vi "Start Tx.vi"(3 "error in (no error)":errorcluster, 5 "Cluster":T1) -> (0 "error out":errorcluster)   [LabVIEW 2015, in "QCA_DUT_Func.lvlib"]
doc: "DLL_QMSL_AEROFLEX void _stdcall StartTx(int txMode,int channel,int rateBitIndex0,int wlanMode,int pktLen0,int txChain0,int shortGuard,int numPackets,int broadcast,int flags,int gainIdx,int dacGain,int paConfig,int tpcm);"
uses:
  QCA_DUT_Func.lvlib
  QCA_DUT_Func.dll
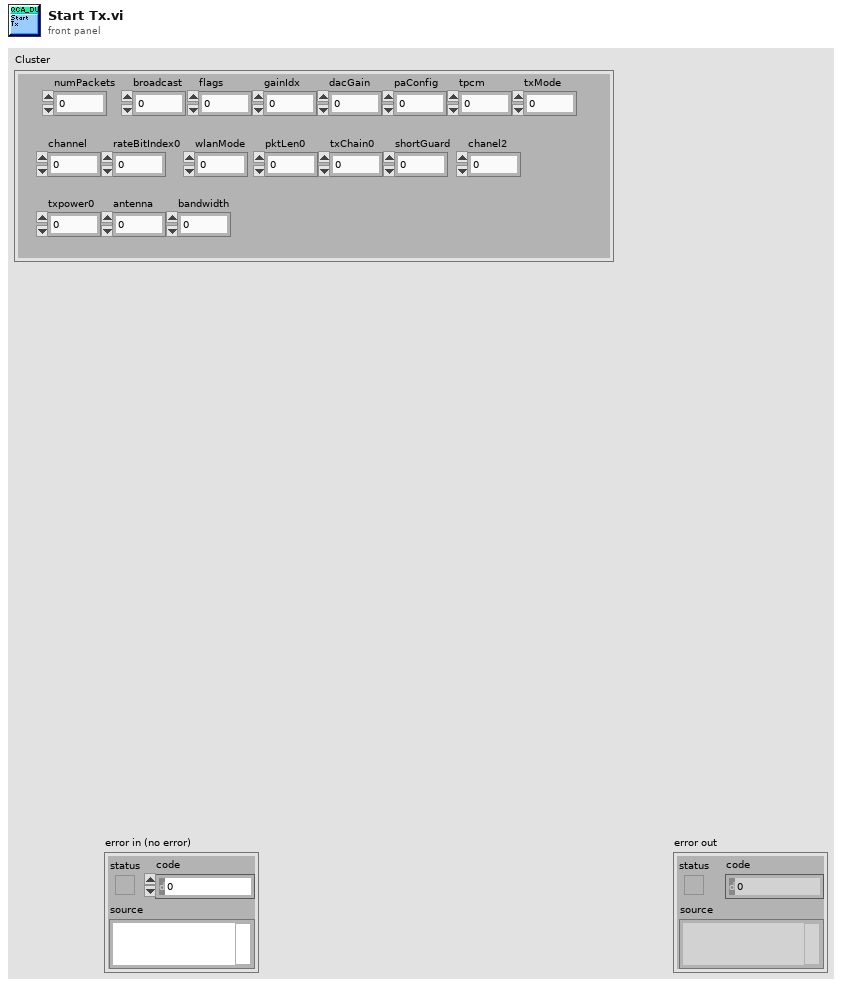
[diagram p1: front panel]
types:
  T1 = cluster{"numPackets":i32, "broadcast":i32, "flags":i32, "gainIdx":i32, "dacGain":i32, "paConfig":i32, "tpcm":i32, "txMode":i32, "channel":i32, "rateBitIndex0":i32, "wlanMode":i32, "pktLen0":i32, "txChain0":i32, "shortGuard":i32, "chanel2":i32, "txpower0":dbl, "antenna":i32, "bandwidth":i32}
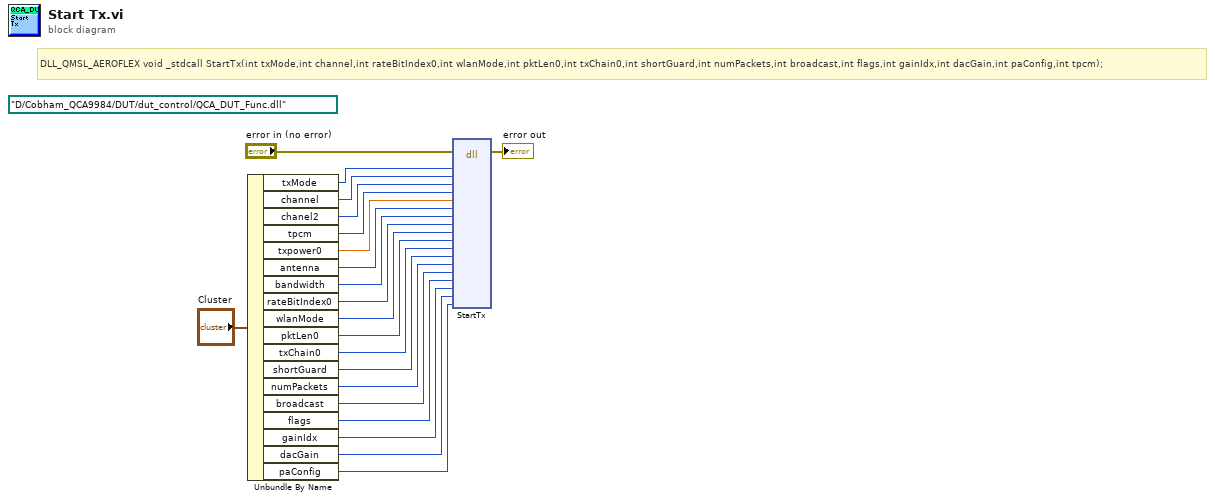
[diagram p0: block diagram]
diagram:
  (unwired) path "D:/Cobham_QCA9984/DUT/dut_control/QCA_DUT_Func.dll" ("path in")
  # "DLL_QMSL_AEROFLEX void _stdcall StartTx(int txMode,int channel,int rateBitIndex0,int wlanMode,int pktLen0,int txChain0,int shortGuard,int numPackets,int broadcast,int flags,int gainIdx,int dacGain,int paConfig,int tpcm);"
  n1 = Unbundle By Name("Cluster") -> ("txMode"=w18:i32, "channel"=w17:i32, "chanel2"=w16:i32, "tpcm"=w15:i32, "txpower0"=w14:dbl, "antenna"=w13:i32, "bandwidth"=w12:i32, "rateBitIndex0"=w11:i32, "wlanMode"=w10:i32, "pktLen0"=w9:i32, "txChain0"=w8:i32, "shortGuard"=w7:i32, "numPackets"=w6:i32, "broadcast"=w5:i32, "flags"=w4:i32, "gainIdx"=w3:i32, "dacGain"=w2:i32, "paConfig"=w1:i32)
  n2 = dll-call lib="D:/4-Up-WLAN-Test-System/DUT Control/DUT/dut_control/QCA_DUT_Func.dll" fn="StartTx"(error in="error in (no error)", "txMode"=w18, "channel"=w17, "chanel2"=w16, "tpcm"=w15, "txpower0"=w14, "antenna"=w13, "bandwidth"=w12, "rateBitIndex0"=w11, "wlanMode"=w10, "pktLen0"=w9, "txChain0"=w8, "shortGuard"=w7, "numPackets"=w6, "broadcast"=w5, "flags"=w4, "gainIdx"=w3, "dacGain"=w2, "paConfig"=w1) -> (error out=→"error out":errorcluster)  [unwired: 21 in, 1 out]
